vi "Image Type to bytes per pixel.vi"(11 "Image Type":T1 items=["Grayscale (U8)", "Grayscale (I16)", "Grayscale (SGL)", "Complex (CSG)", "RGB (U32)", "HSL (U32)", "RGB (U64)", "Grayscale (U16)"]) -> (3 "Bytes per Pixel":u32)   [LabVIEW 2013, in "KLB.lvlib"]
doc: "Takes IMAQ Image Type and gives number of bytes per pixel\n\nUseful for memory size calculations"
uses:
  KLB.lvlib
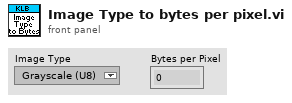
[diagram p1: front panel]
types:
  T1 = typedef "Image Type" = u32
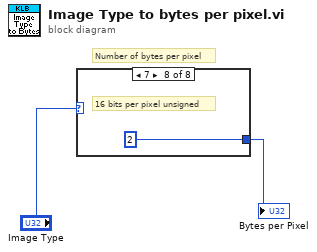
[diagram p0: block diagram]
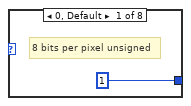
[diagram p2: hidden frame]
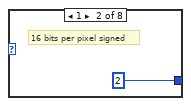
[diagram p3: hidden frame]
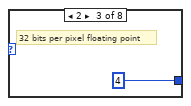
[diagram p4: hidden frame]
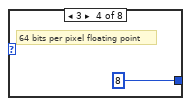
[diagram p5: hidden frame]
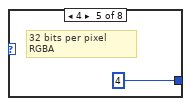
[diagram p6: hidden frame]
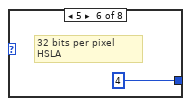
[diagram p7: hidden frame]
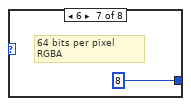
[diagram p8: hidden frame]
diagram:
  # "Number of bytes per pixel"
  n1 = case shown="7" "Image Type" {
    tunnel: [u32 1 u32 2 u32 4 u32 8 u32 4 u32 4 u32 8 u32 2] -> w2
    frame 0, Default {
      # "8 bits per pixel unsigned"
    }
    frame 1 {
      # "16 bits per pixel signed"
    }
    frame 2 {
      # "32 bits per pixel floating point"
    }
    frame 3 {
      # "64 bits per pixel floating point"
    }
    frame 4 {
      # "32 bits per pixel RGBA"
    }
    frame 5 {
      # "32 bits per pixel HSLA"
    }
    frame 6 {
      # "64 bits per pixel RGBA"
    }
    frame 7 {
      # "16 bits per pixel unsigned"
    }
  }
  "Bytes per Pixel" <- w2
